vi "启动参数设置.vi"() -> ()   [LabVIEW 2016, in "斯坦道氨氮.lvlib"]
uses:
  <vilib>/Utility/miscctls.llb/LVPointTypeDef.ctl
  <vilib>/Utility/config.llb/NI_LVConfig.lvlib
panel:
  in  "启动参数":T1
  in  "取消":bool
  in  "确认":bool
  # "请选择启动参数"
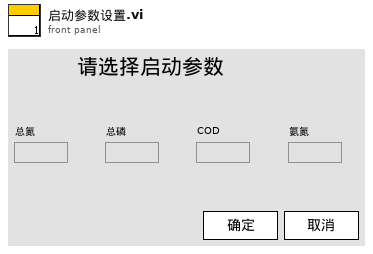
[diagram p1: front panel]
types:
  T1 = cluster{"COD":bool, "氨氮":bool, "总氮":bool, "总磷":bool}
  T2 = typedef "LVPointTypeDef.ctl" = cluster{"Horizontal":i16, "Vertical":i16}
  T3 = typedef "NI_LVConfig.lvlib/Config Data RefNum.ctl" = refnum<k1>
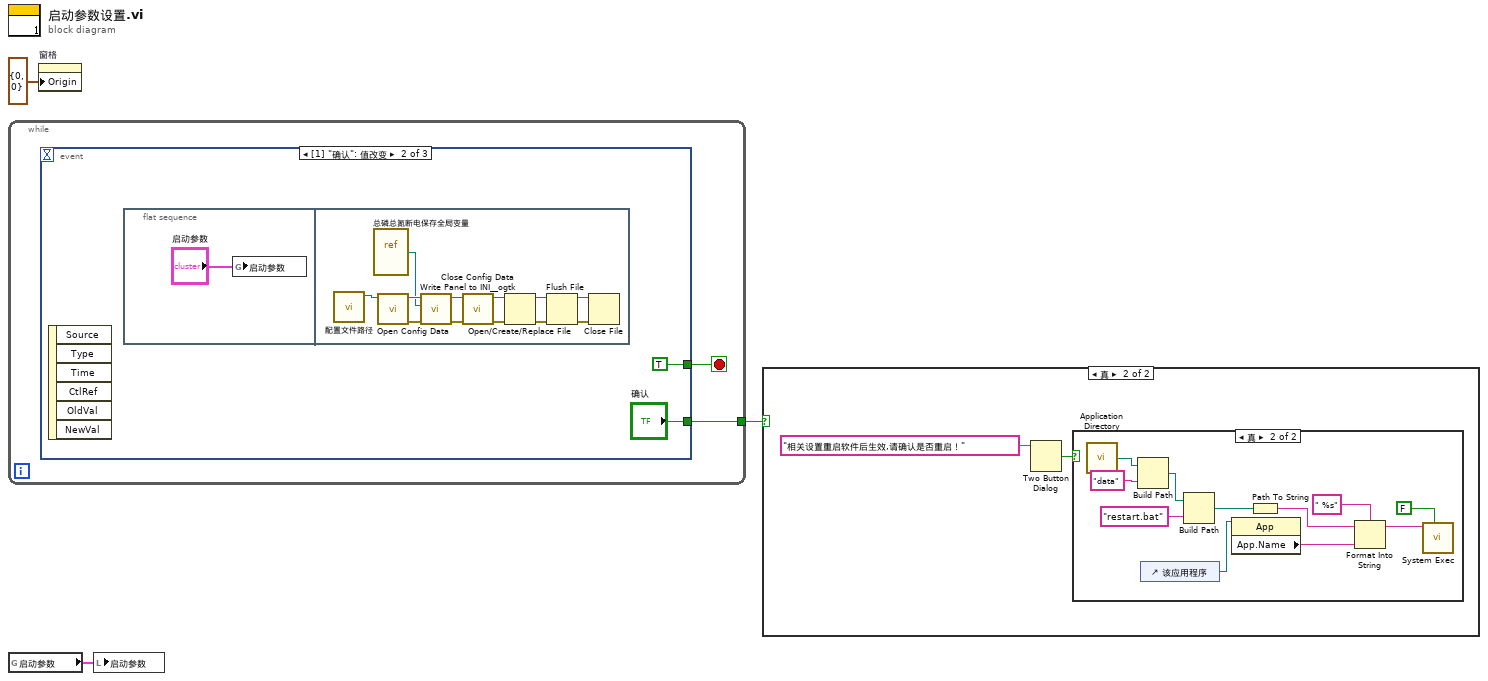
[diagram p0: block diagram]
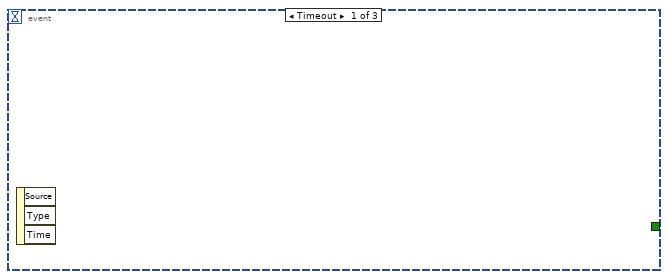
[diagram p4: hidden frame]
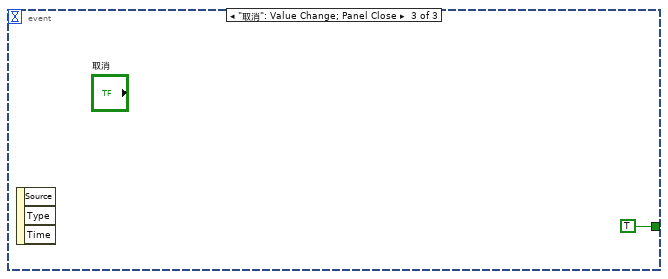
[diagram p5: hidden frame]
diagram:
  n1 = while {
    tunnel: [w4] -> w1
    stop <- w5 stop-if-true
    n2 = event shown="[1] \"确认\": 值改变" {
      selector: _ -> [_ _ _]
      dyn-events: _ -> [_ _ _]
      timeout: _ -> [_ _ _]
      tunnel: [_ TRUE TRUE] -> w5
      tunnel: [_ "确认" _] -> w4
      event Timeout {
        n3 = event-data() -> ()  [unwired: 1 in, 3 out]
      }
      event "确认": Value Change {
        n4 = event-data() -> ()  [unwired: 1 in, 6 out]
        n5 = flat-sequence {
          frame #0 {
            n6 = global write "总磷总氮断电保存全局变量.vi" "启动参数"("启动参数") -> ()
          }
          frame #1 {
            n7 = call "配置文件路径.vi"() -> ("appended path"=w9:path)  [unwired: 11 in]
            n8 = vi-ref "总磷总氮断电保存全局变量.vi"() -> (w19:refnum<vi>)
            n9 = call <vilib>:"Open Config Data.vi"("configuration file path"=w9) -> ("error out"=w17:errorcluster, "refnum"=w20:T3)  [unwired: 8 in, 1 out]
            n10 = call <userlib>:"Write Panel to INI__ogtk.vi"("error in (no error)"=w17, "VI ref"=w19, "refnum"=w20) -> ("error out"=w16:errorcluster, "refnum out"=w18:T3)  [unwired: 7 in]
            n11 = call <vilib>:"Close Config Data.vi"("error in (no error)"=w16, "refnum"=w18) -> ("error out"=w11:errorcluster, "file path"=w10:path)  [unwired: 8 in]
            n12 = Open/Create/Replace File(file path (use dialog)=w10, error in=w11) -> (refnum out=w14:refnum<file>, error out=w15:errorcluster)  [unwired: 4 in, 1 out]
            n13 = Flush File(refnum=w14, error in=w15) -> (refnum out=w13:refnum<file>, error out=w12:errorcluster)
            n14 = Close File(refnum=w13, error in=w12) -> ()  [unwired: 2 out]
          }
        }
      }
      event "取消": Value Change; Panel Close {
        n15 = event-data() -> ()  [unwired: 1 in, 3 out]
      }
    }
  }
  n16 = global read "总磷总氮断电保存全局变量.vi" "启动参数"() -> (w2:T1)
  n17 = property on="窗格" class="Pane"("Origin"=T2 {"Horizontal"=0, "Vertical"=0} ("原点")) -> ()  [unwired: 2 in, 2 out]
  n18 = local write "启动参数"(w2) -> ()
  n19 = case shown="真" w1 {
    frame False {
    }
    frame True {
      n20 = Two Button Dialog(message="相关设置重启软件后生效,请确认是否重启！" ("按钮名称（“确定”）")) -> (T button?=w22:bool)  [unwired: 2 in]
      n21 = case shown="真" w22 {
        frame False {
        }
        frame True {
          n22 = call <vilib>:"Application Directory.vi"() -> ("Application Directory"=w25:path)
          n23 = Build Path(base path=w25, name or relative path="data" ("名称或相对路径")) -> (appended path=w27:path)
          n24 = control-ref of="该应用程序"() -> (w24:refnum<vi>)
          n25 = Build Path(base path=w27, name or relative path="restart.bat" ("名称或相对路径")) -> (appended path=w29:path)
          n26 = property class="App"(reference=w24) -> ("App.Name"=w32:string)  [unwired: 1 in, 2 out]
          n27 = Path To String(path=w29) -> (string=w30:string)
          n28 = Format Into String(format string=" %s" ("格式字符串"), initial string=w30, w32) -> (resulting string=w33:string)  [unwired: 1 in, 1 out]
          n29 = call <vilib>:"System Exec.vi"("wait until completion? (T)"=FALSE, "command line"=w33) -> ()  [unwired: 6 in, 4 out]
        }
      }
    }
  }
